vi "Hydrosonic_Manual.vi"() -> ()   [LabVIEW 2020]
panel:
  in  "Mode":T1(ring)
  out "Tranducer Value":dbl format="%.2f"
  out "Transducer Error Info":string
  in  "Set Tranducer Value":T2(ring)
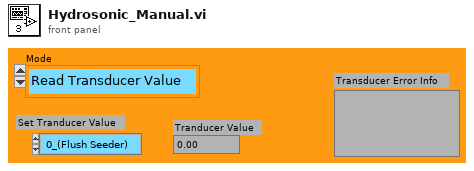
[diagram p1: front panel]
types:
  T1 = enum16{"Read Transducer Value", "Set Transducer value"}
  T2 = enum16{" 0_(Flush Seeder)", "5_(No Seeding)", "10", "20", "30", "40", "50", "60", "70", "80", "90", "100"}
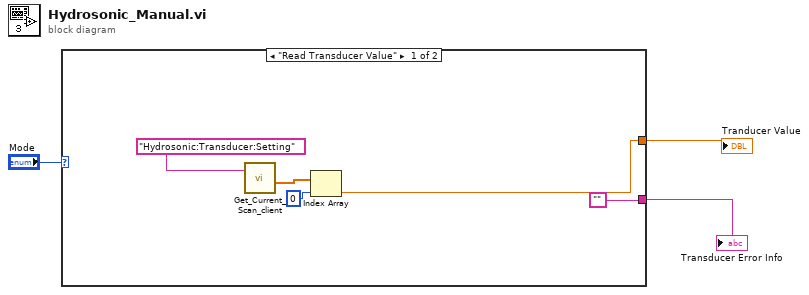
[diagram p0: block diagram]
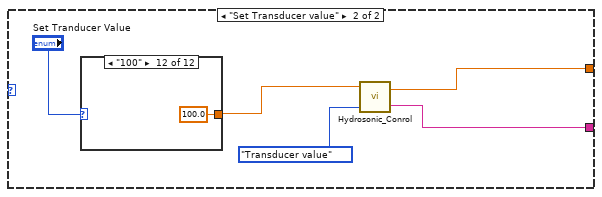
[diagram p2: hidden frame]
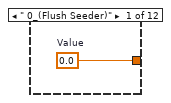
[diagram p3: hidden frame]
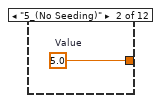
[diagram p4: hidden frame]
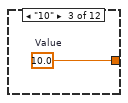
[diagram p5: hidden frame]
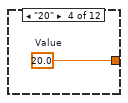
[diagram p6: hidden frame]
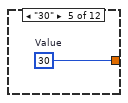
[diagram p7: hidden frame]
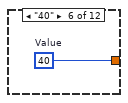
[diagram p8: hidden frame]
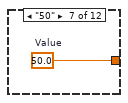
[diagram p9: hidden frame]
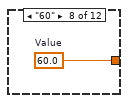
[diagram p10: hidden frame]
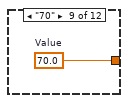
[diagram p11: hidden frame]
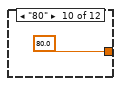
[diagram p12: hidden frame]
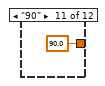
[diagram p13: hidden frame]
diagram:
  n1 = case shown="\"Read Transducer Value\"" "Mode" {
    tunnel: [w5 w10] -> w3
    tunnel: ["" w9] -> w2
    frame "Read Transducer Value" {
      n2 = call "Get_Current_Scan_client.vi"("singleChannel"="Hydrosonic:Transducer:Setting") -> ("Numerical Values"=w8:dbl[])  [unwired: 2 in, 2 out]
      n3 = Index Array(array=w8, index=0) -> (element=w5:dbl)
    }
    frame "Set Transducer value" {
      n4 = case shown="\"100\"" "Set Tranducer Value" {
        tunnel: [w14 w15 w16 w17 w18 w19 w20 w21 w22 80.0 90.0 ("Value") 100.0 ("Value")] -> w11
        frame " 0_(Flush Seeder)" {
          w14 = 0.0  # Value
        }
        frame "5_(No Seeding)" {
          w15 = 5.0  # Value
        }
        frame "10" {
          w16 = 10.0  # Value
        }
        frame "20" {
          w17 = 20.0  # Value
        }
        frame "30" {
          w18 = 30  # Value
        }
        frame "40" {
          w19 = 40  # Value
        }
        frame "50" {
          w20 = 50.0  # Value
        }
        frame "60" {
          w21 = 60.0  # Value
        }
        frame "70" {
          w22 = 70.0  # Value
        }
        frame "80" {
        }
        frame "90" {
        }
        frame "100" {
        }
      }
      n5 = call "Hydrosonic_Conrol.vi"("Input Mode"=enum16{"Desired Frequency", "Transducer value"}."Transducer value", "Desired Value"=w11) -> ("Error Info"=w9:string, "Set output"=w10:dbl)  [unwired: 2 in]
    }
  }
  "Transducer Error Info" <- w2
  "Tranducer Value" <- w3
